vi "Pe.vi"() -> ()   [LabVIEW 2013]
uses:
  <vilib>/gmath/NI_Gmath.lvlib
panel:
  in  "M":dbl
  out "Numeric":dbl
  in  "SNR":dbl
  in  "Knob":dbl(knob) scale=0.0..10.0
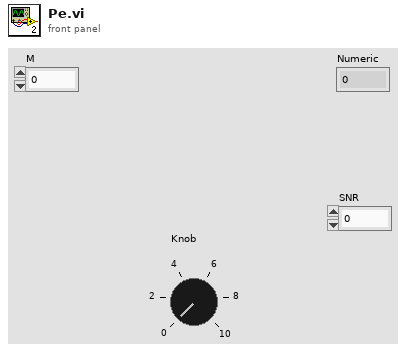
[diagram p1: front panel]
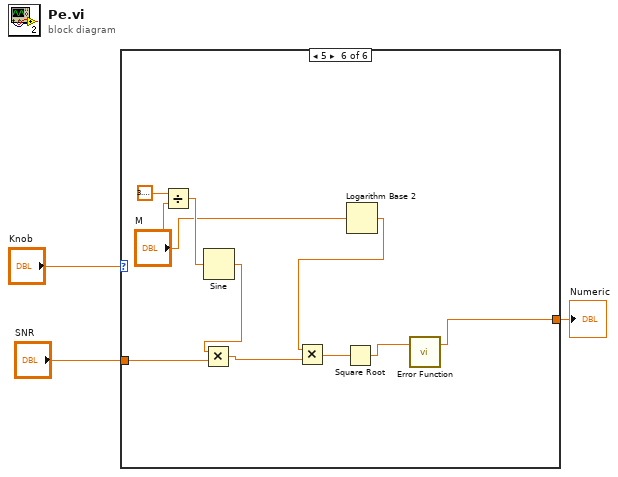
[diagram p0: block diagram]
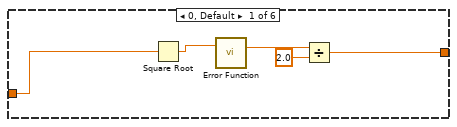
[diagram p2: hidden frame]
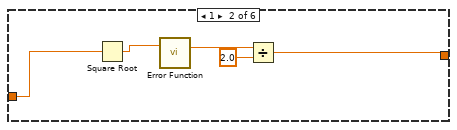
[diagram p3: hidden frame]
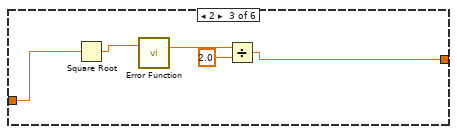
[diagram p4: hidden frame]
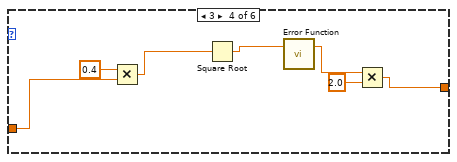
[diagram p5: hidden frame]
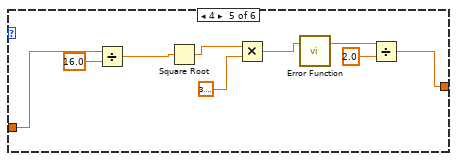
[diagram p6: hidden frame]
diagram:
  n1 = case shown="5" "Knob" {
    tunnel: "SNR" -> [w8 w10 w15 w25 w34 w44]
    tunnel: [w4 w9 w14 w19 w30 w35] -> w1
    frame 0, Default {
      n2 = Square Root(x=w8) -> (sqrt(x)=w7:dbl)
      n3 = call <vilib>:"Error Function.vi"("x"=w7) -> ("erf(x)"=w6:dbl)  [unwired: 2 in]
      n4 = Divide(x=w6, y=2.0) -> (x/y=w4:dbl)
    }
    frame 1 {
      n5 = Square Root(x=w10) -> (sqrt(x)=w13:dbl)
      n6 = call <vilib>:"Error Function.vi"("x"=w13) -> ("erf(x)"=w12:dbl)  [unwired: 2 in]
      n7 = Divide(x=w12, y=2.0) -> (x/y=w9:dbl)
    }
    frame 2 {
      n8 = Square Root(x=w15) -> (sqrt(x)=w18:dbl)
      n9 = call <vilib>:"Error Function.vi"("x"=w18) -> ("erf(x)"=w17:dbl)  [unwired: 2 in]
      n10 = Divide(x=w17, y=2.0) -> (x/y=w14:dbl)
    }
    frame 3 {
      n11 = Multiply(x=0.4, y=w25) -> (x*y=w23:dbl)
      n12 = Square Root(x=w23) -> (sqrt(x)=w22:dbl)
      n13 = call <vilib>:"Error Function.vi"("x"=w22) -> ("erf(x)"=w21:dbl)  [unwired: 2 in]
      n14 = Multiply(x=w21, y=2.0) -> (x*y=w19:dbl)
    }
    frame 4 {
      n15 = Divide(x=w34, y=16.0) -> (x/y=w29:dbl)
      n16 = Square Root(x=w29) -> (sqrt(x)=w28:dbl)
      n17 = Multiply(x=w28, y=3.141592653589793) -> (x*y=w26:dbl)
      n18 = call <vilib>:"Error Function.vi"("x"=w26) -> ("erf(x)"=w32:dbl)  [unwired: 2 in]
      n19 = Divide(x=w32, y=2.0) -> (x/y=w30:dbl)
    }
    frame 5 {
      n20 = Divide(x=3.141592653589793, y="M") -> (x/y=w42:dbl)
      n21 = Sine(x=w42) -> (sin(x)=w41:dbl)
      n22 = Multiply(x=w41, y=w44) -> (x*y=w40:dbl)
      n23 = Logarithm Base 2(1:"M") -> (0:w38:dbl)
      n24 = Multiply(x=w38, y=w40) -> (x*y=w37:dbl)
      n25 = Square Root(x=w37) -> (sqrt(x)=w36:dbl)
      n26 = call <vilib>:"Error Function.vi"("x"=w36) -> ("erf(x)"=w35:dbl)  [unwired: 2 in]
    }
  }
  "Numeric" <- w1
